vi "PDF-Add To Catalog.vi"(0 "catalog in":T1, 5 "Title":string, 7 "VI reference":refnum<vi>, 11 "error in (no error)":errorcluster) -> (4 "catalog out":T1, 15 "error out":errorcluster)   [LabVIEW 2020]
uses:
  PDF-Catalog.ctl
  <vilib>/Exaprom PDF/LV Class/PDF Report Class/PDF Report Class.lvclass
  <vilib>/Exaprom PDF/Controls/Image Controls/Image alignment and position.ctl
  <vilib>/Exaprom PDF/Controls/Image Controls/Image aligment.ctl
  <vilib>/Exaprom PDF/Controls/Image Controls/Image border.ctl
  <vilib>/Exaprom PDF/Controls/Initialization Controls/Defaut Paragraphe and Line Spacing.ctl
  <vilib>/Exaprom PDF/Controls/Text Controls/Texte alignement.ctl
  <vilib>/Exaprom PDF/Controls/Text Controls/Line spacing.ctl
  <vilib>/Exaprom PDF/Controls/Font Controls/Font complete cluster.ctl
  <vilib>/Exaprom PDF/Controls/Font Controls/Font size.ctl
  <vilib>/Exaprom PDF/Controls/Font Controls/Font color.ctl
  <vilib>/Exaprom PDF/Controls/Font Controls/Type and encoding.ctl
  <vilib>/Exaprom PDF/Controls/Text Controls/Unicode/Type and run direction.ctl
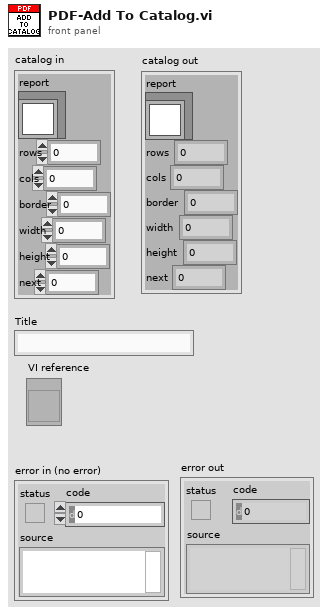
[diagram p1: front panel]
types:
  T1 = typedef "PDF-Catalog.ctl" = cluster{"report":refnum<class "PDF Report Class.lvclass">, "rows":i32, "cols":i32, "border":dbl, "width":dbl, "height":dbl, "next":i32}
  T2 = typedef "Image border.ctl" = cluster{"Show?":bool, "Thickness (point)":sgl, "Color":u32}
  T3 = typedef "Image alignment and position.ctl" = cluster{"Alignment":T4, "X ":sgl, "Y":sgl, "Indentation":sgl}
  T4 = typedef "Image aligment.ctl" = enum16{"Absolute (X,Y)", "Left", "Center", "Right", "Left (textwrap)", "Right (textwrap)"}
  T5 = typedef "Font complete cluster.ctl" = cluster{"Name":string, "Size":T6, "Color":T7, "Style":cluster{"Bold":bool, "Italic":bool, "Underline":bool, "Strikeout":bool}, "Type":T8}
  T6 = typedef "Font size.ctl" = sgl
  T7 = typedef "Font color.ctl" = u32
  T8 = typedef "Type and encoding.ctl" = cluster{"Type&direction":T9, "Embedded":bool, "Encoding":string}
  T9 = typedef "Type and run direction.ctl" = enum16{"Select", "ASCII", "UTF-16", "UTF-16 (default)", "UTF-16 (LTR)", "UTF-16 (RTL)"}
  T10 = typedef "Defaut Paragraphe and Line Spacing.ctl" = cluster{" Aligment":T11, "Line spacing":T12}
  T11 = typedef "Texte alignement.ctl" = enum16{"Select", "CENTER", "JUSTIFY", "LEFT", "RIGHT"}
  T12 = typedef "Line spacing.ctl" = enum16{"Select", "1.0", "1.5", "2.0"}
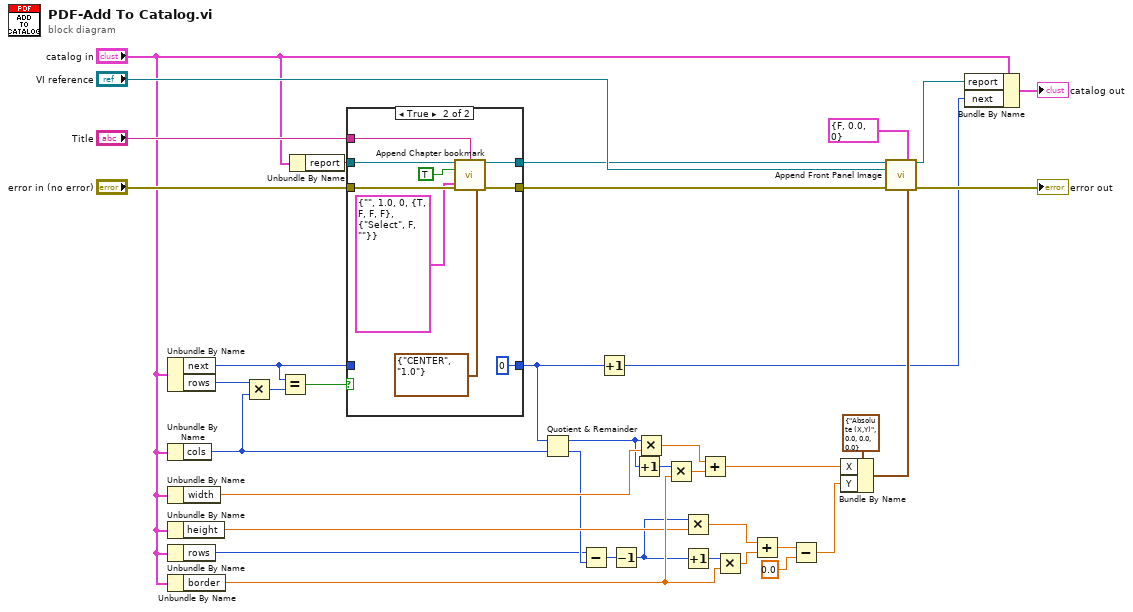
[diagram p0: block diagram]
diagram:
  n1 = Unbundle By Name("catalog in") -> ("next"=w26:i32, "rows"=w5:i32)
  n2 = Unbundle By Name("catalog in") -> ("cols"=w23:i32)
  n3 = Unbundle By Name("catalog in") -> ("width"=w22:dbl)
  n4 = Unbundle By Name("catalog in") -> ("height"=w11:dbl)
  n5 = Unbundle By Name("catalog in") -> ("rows"=w4:i32)
  n6 = Unbundle By Name("catalog in") -> ("border"=w12:dbl)
  n7 = Multiply(x=w5, y=w23) -> (x*y=w28:i32)
  n8 = Equal?(x=w26, y=w28) -> (x = y?=w27:bool)
  n9 = Unbundle By Name("catalog in") -> ("report"=w31:refnum<class "PDF Report Class.lvclass">)
  n10 = case shown="True" w27 {
    tunnel: "Title" -> [_ w50]
    tunnel: [w41 w47] -> w35
    tunnel: [w40 w46] -> w33
    tunnel: "error in (no error)" -> [w40 w45]
    tunnel: w31 -> [w41 w44]
    tunnel: w26 -> [w39 _]
    tunnel: [w39 0] -> w25
    frame False {
    }
    frame True {
      n11 = call <vilib>:"Append Chapter bookmark.vi"("PDF Report"=w44, "Title"=w50, "TriggerNewPage (Chapter)"=TRUE, "error in (no error)"=w45, "Font"=T5 {"Name"="", "Size"=1.0, "Color"=0, "Style"={"Bold"=TRUE, "Italic"=FALSE, "Underline"=FALSE, "Strikeout"=FALSE}, "Type"={"Type&direction"=enum."Select", "Embedded"=FALSE, "Encoding"=""}}, "Title properties"=T10 {" Aligment"=enum."CENTER", "Line spacing"=enum."1.0"}) -> ("PDF Report duplicate"=w47:refnum<class "PDF Report Class.lvclass">, "error out"=w46:errorcluster)  [unwired: 8 in]
    }
  }
  n12 = Quotient & Remainder(x=w25, y=w23) -> (x-y*floor(x/y)=w20:i32, floor(x/y)=w7:i32)
  n13 = Subtract(x=w4, y=w7) -> (x-y=w8:i32)
  n14 = Increment(x=w25) -> (x+1=w10:i32)
  n15 = Decrement(x=w8) -> (x-1=w3:i32)
  n16 = Increment(x=w20) -> (x+1=w21:i32)
  n17 = Multiply(x=w20, y=w22) -> (x*y=w18:dbl)
  n18 = Multiply(x=w21, y=w12) -> (x*y=w19:dbl)
  n19 = Multiply(x=w3, y=w11) -> (x*y=w14:dbl)
  n20 = Increment(x=w3) -> (x+1=w16:i32)
  n21 = Add(x=w18, y=w19) -> (x+y=w17:dbl)
  n22 = Multiply(x=w16, y=w12) -> (x*y=w15:dbl)
  n23 = Add(x=w14, y=w15) -> (x+y=w13:dbl)
  n24 = Subtract(x=w13, y=0.0) -> (x-y=w2:dbl)
  n25 = Bundle By Name(cluster=T3 {"Alignment"=enum."Absolute (X,Y)", "X "=0.0, "Y"=0.0, "Indentation"=0.0} ("Position and indentation"), "X"=w17, "Y"=w2) -> (w24:T3)
  n26 = call <vilib>:"Append Front Panel Image.vi"("PDF Report IN"=w35, "Border"=T2 {"Show?"=FALSE, "Thickness (point)"=0.0, "Color"=0}, "VI reference"="VI reference", "error in (no error)"=w33, "Position and indentation"=w24) -> ("PDF Report OUT"=w30:refnum<class "PDF Report Class.lvclass">, "error out"=→"error out":errorcluster)  [unwired: 9 in]
  n27 = Bundle By Name(cluster="catalog in", "report"=w30, "next"=w10) -> (→"catalog out":T1)
